vi "Degree to Ratation.vi"(9 "Wheel Axel Width (in)":dbl, 10 "Wheel Diameter (in)":dbl, 11 "Rotation (degrees)":dbl) -> (3 "Rotations needed":dbl)   [LabVIEW 2014]
doc: "Converts a desired turn amount in degrees based on robot dimensions to wheel rotations."
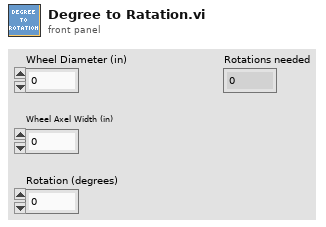
[diagram p1: front panel]
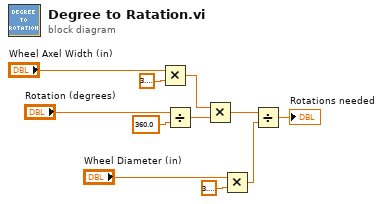
[diagram p0: block diagram]
diagram:
  n1 = Multiply(x="Wheel Axel Width (in)", y=3.141592653589793) -> (x*y=w5:dbl)
  n2 = Divide(x="Rotation (degrees)", y=360.0) -> (x/y=w4:dbl)
  n3 = Multiply(x=w5, y=w4) -> (x*y=w3:dbl)
  n4 = Multiply(x="Wheel Diameter (in)", y=3.141592653589793) -> (x*y=w2:dbl)
  n5 = Divide(x=w3, y=w2) -> (x/y=→"Rotations needed":dbl)
